vi "nchFFT.vi"(4 "1ch":dbl[](array[numeric]) caption="X1", 5 "频率":dbl) -> (0 "频谱图":dbl[](graph), 2 "幅度值1":dbl)   [LabVIEW 2014]
uses:
  <vilib>/Analysis/2dsp.llb/Real FFT.vi
  <vilib>/Analysis/NI_AALPro.lvlib
panel:
  in  "8ch":dbl[](array[numeric]) caption="X8"
  out "幅度值8":dbl
  out "频谱图 8":dbl[](graph)
  in  "7ch":dbl[](array[numeric]) caption="X7"
  out "幅度值7":dbl
  out "频谱图 7":dbl[](graph)
  in  "6ch":dbl[](array[numeric]) caption="X6"
  out "幅度值6":dbl
  out "频谱图 6":dbl[](graph)
  in  "5ch":dbl[](array[numeric]) caption="X5"
  out "幅度值5":dbl
  out "频谱图 5":dbl[](graph)
  in  "4ch":dbl[](array[numeric]) caption="X4"
  out "幅度值4":dbl
  out "频谱图 4":dbl[](graph)
  in  "3ch":dbl[](array[numeric]) caption="X3"
  out "幅度值3":dbl
  out "频谱图 3":dbl[](graph)
  in  "2ch":dbl[](array[numeric]) caption="X2"
  out "幅度值2":dbl
  out "频谱图 2":dbl[](graph)
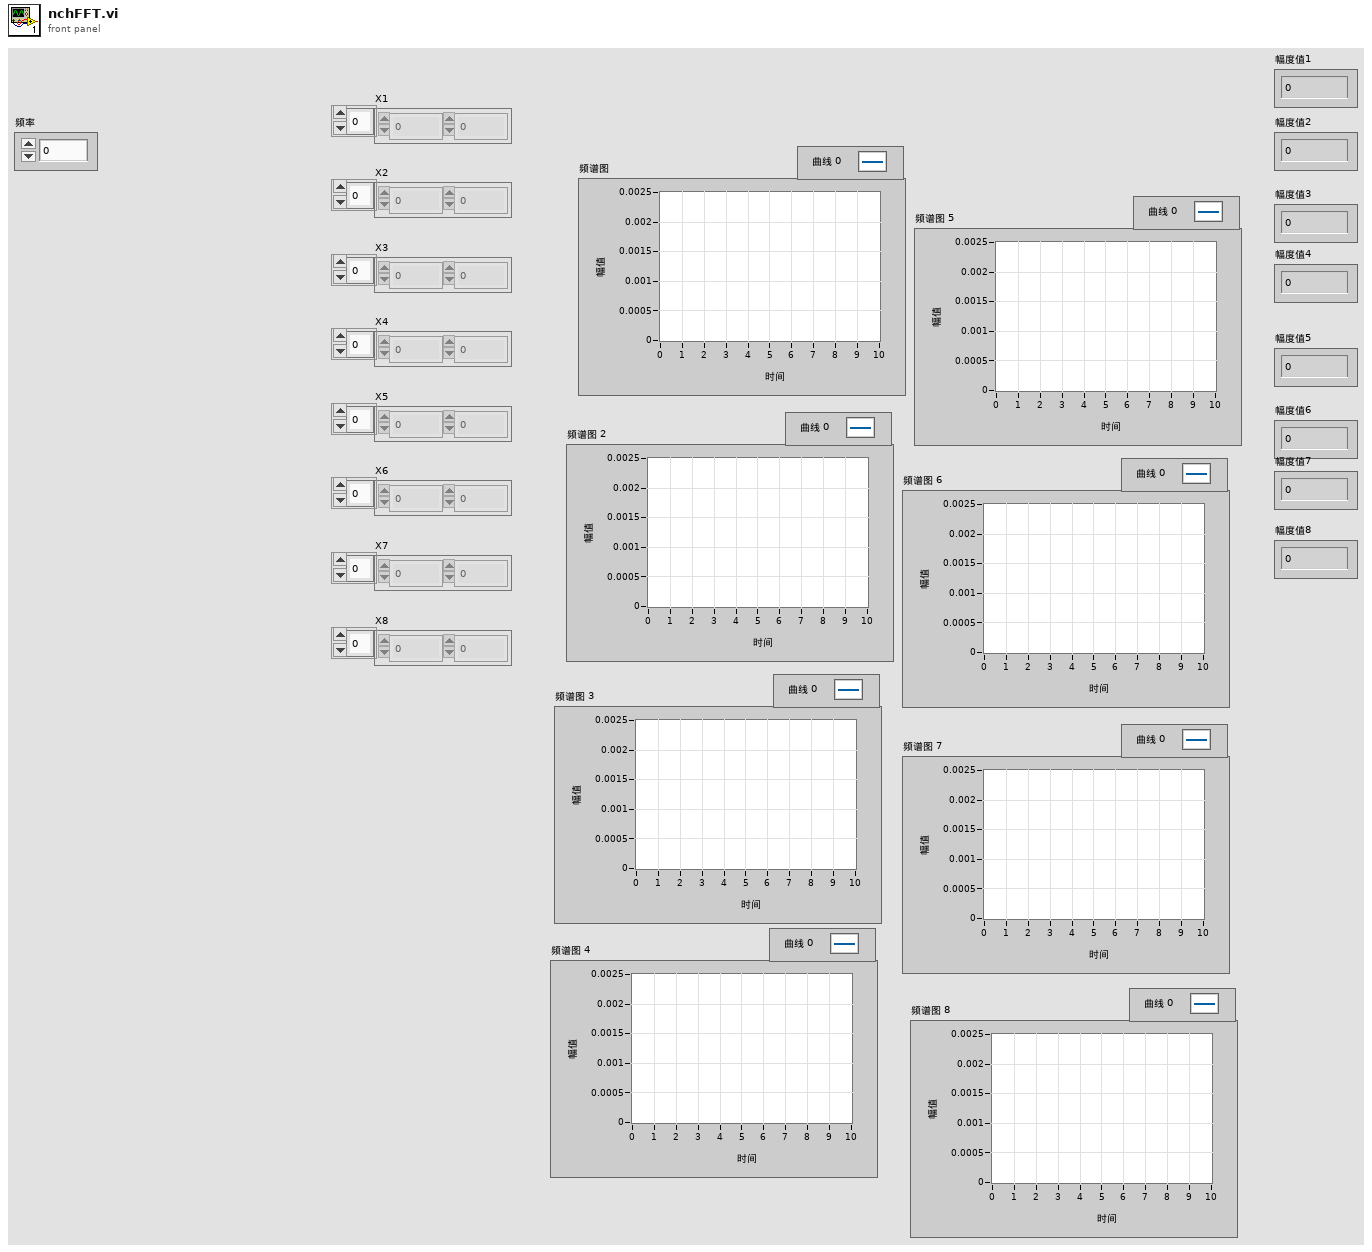
[diagram p1: front panel]
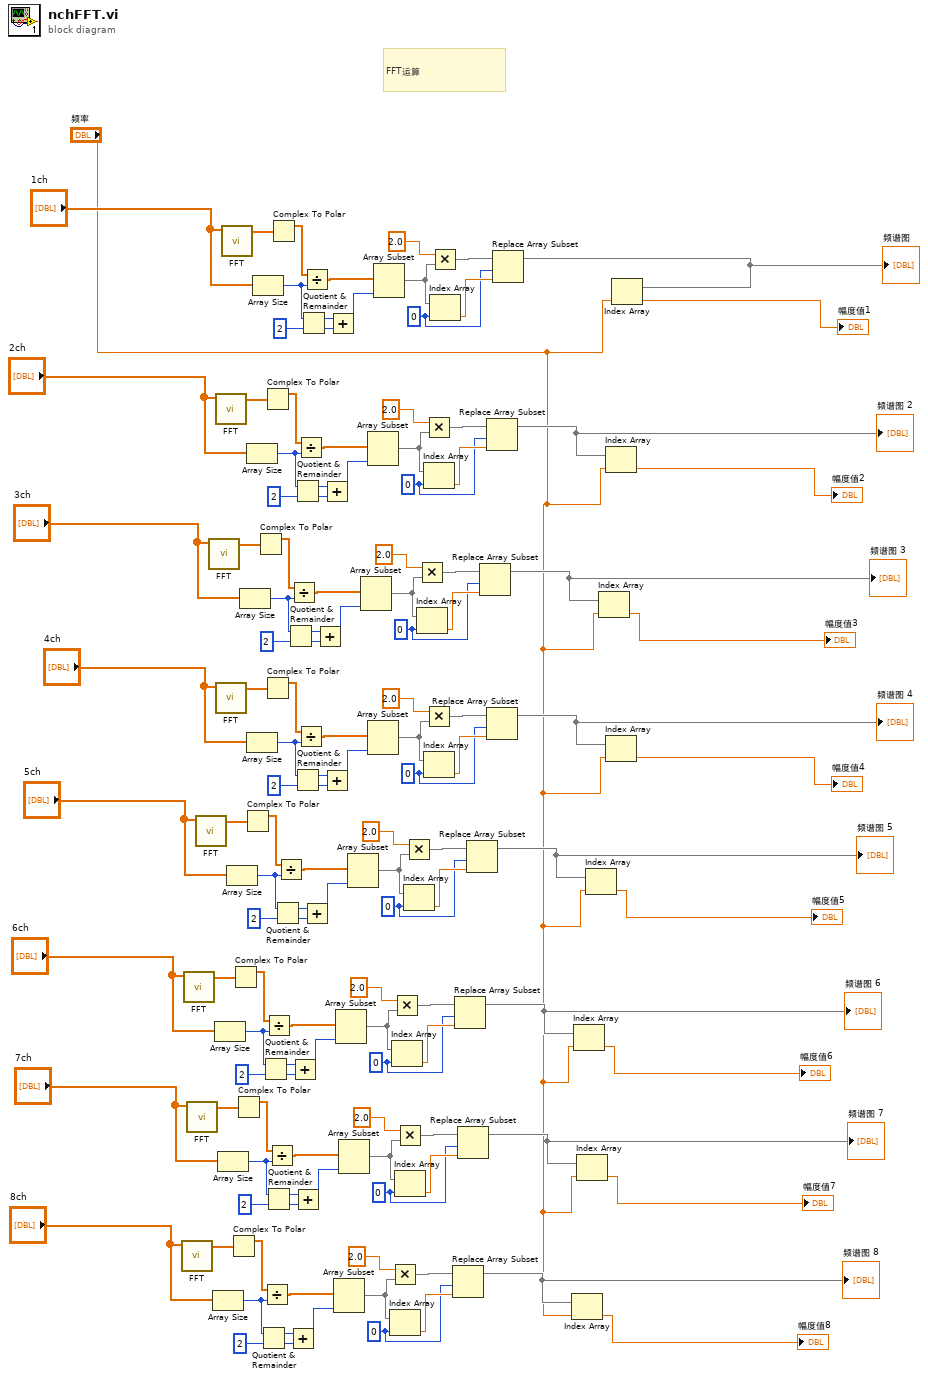
[diagram p0: block diagram]
diagram:
  w8 = 0 ("索引")
  w24 = 0 ("索引")
  w40 = 0 ("索引")
  w56 = 0 ("索引")
  w72 = 0 ("索引")
  w88 = 0 ("索引")
  w104 = 0 ("索引")
  w120 = 0 ("索引")
  # "FFT运算"
  n1 = call-poly <vilib>:"FFT.vi"("X"="8ch") -> ("FFT {X}"=w17:cdb[])  [unwired: 9 in, 1 out]
  n2 = call-poly <vilib>:"FFT.vi"("X"="6ch") -> ("FFT {X}"=w49:cdb[])  [unwired: 9 in, 1 out]
  n3 = call-poly <vilib>:"FFT.vi"("X"="7ch") -> ("FFT {X}"=w33:cdb[])  [unwired: 9 in, 1 out]
  n4 = call-poly <vilib>:"FFT.vi"("X"="5ch") -> ("FFT {X}"=w65:cdb[])  [unwired: 9 in, 1 out]
  n5 = call-poly <vilib>:"FFT.vi"("X"="3ch") -> ("FFT {X}"=w97:cdb[])  [unwired: 9 in, 1 out]
  n6 = Array Size(array="8ch") -> (size(s)=w6:i32)
  n7 = Array Size(array="6ch") -> (size(s)=w38:i32)
  n8 = call-poly <vilib>:"FFT.vi"("X"="2ch") -> ("FFT {X}"=w113:cdb[])  [unwired: 9 in, 1 out]
  n9 = call-poly <vilib>:"FFT.vi"("X"="4ch") -> ("FFT {X}"=w81:cdb[])  [unwired: 9 in, 1 out]
  n10 = Array Size(array="7ch") -> (size(s)=w22:i32)
  n11 = call-poly <vilib>:"FFT.vi"("X"="1ch") -> ("FFT {X}"=w129:cdb[])  [unwired: 9 in, 1 out]
  n12 = Array Size(array="5ch") -> (size(s)=w54:i32)
  n13 = Complex To Polar(r * e^(i*theta)=w17) -> (r=w16:dbl[])  [unwired: 1 out]
  n14 = Complex To Polar(r * e^(i*theta)=w49) -> (r=w48:dbl[])  [unwired: 1 out]
  n15 = Complex To Polar(r * e^(i*theta)=w33) -> (r=w32:dbl[])  [unwired: 1 out]
  n16 = Array Size(array="3ch") -> (size(s)=w86:i32)
  n17 = Complex To Polar(r * e^(i*theta)=w65) -> (r=w64:dbl[])  [unwired: 1 out]
  n18 = Array Size(array="2ch") -> (size(s)=w102:i32)
  n19 = Array Size(array="4ch") -> (size(s)=w70:i32)
  n20 = Array Size(array="1ch") -> (size(s)=w118:i32)
  n21 = Complex To Polar(r * e^(i*theta)=w97) -> (r=w96:dbl[])  [unwired: 1 out]
  n22 = Quotient & Remainder(x=w6, y=2) -> (x-y*floor(x/y)=w14:i32, floor(x/y)=w15:i32)
  n23 = Quotient & Remainder(x=w38, y=2) -> (x-y*floor(x/y)=w46:i32, floor(x/y)=w47:i32)
  n24 = Divide(x=w16, y=w6) -> (x/y=w7:dbl[])
  n25 = Complex To Polar(r * e^(i*theta)=w113) -> (r=w112:dbl[])  [unwired: 1 out]
  n26 = Complex To Polar(r * e^(i*theta)=w81) -> (r=w80:dbl[])  [unwired: 1 out]
  n27 = Divide(x=w48, y=w38) -> (x/y=w39:dbl[])
  n28 = Quotient & Remainder(x=w22, y=2) -> (x-y*floor(x/y)=w30:i32, floor(x/y)=w31:i32)
  n29 = Divide(x=w32, y=w22) -> (x/y=w23:dbl[])
  n30 = Complex To Polar(r * e^(i*theta)=w129) -> (r=w128:dbl[])  [unwired: 1 out]
  n31 = Quotient & Remainder(x=w54, y=2) -> (x-y*floor(x/y)=w62:i32, floor(x/y)=w63:i32)
  n32 = Divide(x=w64, y=w54) -> (x/y=w55:dbl[])
  n33 = Quotient & Remainder(x=w86, y=2) -> (x-y*floor(x/y)=w94:i32, floor(x/y)=w95:i32)
  n34 = Add(x=w14, y=w15) -> (x+y=w13:i32)
  n35 = Divide(x=w96, y=w86) -> (x/y=w87:dbl[])
  n36 = Add(x=w46, y=w47) -> (x+y=w45:i32)
  n37 = Quotient & Remainder(x=w102, y=2) -> (x-y*floor(x/y)=w110:i32, floor(x/y)=w111:i32)
  n38 = Quotient & Remainder(x=w70, y=2) -> (x-y*floor(x/y)=w78:i32, floor(x/y)=w79:i32)
  n39 = Add(x=w30, y=w31) -> (x+y=w29:i32)
  n40 = Divide(x=w112, y=w102) -> (x/y=w103:dbl[])
  n41 = Divide(x=w80, y=w70) -> (x/y=w71:dbl[])
  n42 = Quotient & Remainder(x=w118, y=2) -> (x-y*floor(x/y)=w126:i32, floor(x/y)=w127:i32)
  n43 = Divide(x=w128, y=w118) -> (x/y=w119:dbl[])
  n44 = Add(x=w62, y=w63) -> (x+y=w61:i32)
  n45 = Add(x=w94, y=w95) -> (x+y=w93:i32)
  n46 = Add(x=w110, y=w111) -> (x+y=w109:i32)
  n47 = Add(x=w78, y=w79) -> (x+y=w77:i32)
  n48 = Add(x=w126, y=w127) -> (x+y=w125:i32)
  n49 = Array Subset(array=w7, length=w13) -> (w11:dbl[])  [unwired: 1 in]
  n50 = Array Subset(array=w39, length=w45) -> (w43:dbl[])  [unwired: 1 in]
  n51 = Array Subset(array=w23, length=w29) -> (w27:dbl[])  [unwired: 1 in]
  n52 = Array Subset(array=w55, length=w61) -> (w59:dbl[])  [unwired: 1 in]
  n53 = Array Subset(array=w87, length=w93) -> (w91:dbl[])  [unwired: 1 in]
  n54 = Array Subset(array=w103, length=w109) -> (w107:dbl[])  [unwired: 1 in]
  n55 = Array Subset(array=w71, length=w77) -> (w75:dbl[])  [unwired: 1 in]
  n56 = Array Subset(array=w119, length=w125) -> (w123:dbl[])  [unwired: 1 in]
  n57 = Multiply(x=2.0, y=w11) -> (x*y=w9:dbl[])
  n58 = Index Array(array=w11, index=w8) -> (element=w10:dbl)
  n59 = Multiply(x=2.0, y=w43) -> (x*y=w41:dbl[])
  n60 = Index Array(array=w43, index=w40) -> (element=w42:dbl)
  n61 = Multiply(x=2.0, y=w27) -> (x*y=w25:dbl[])
  n62 = Index Array(array=w27, index=w24) -> (element=w26:dbl)
  n63 = Multiply(x=2.0, y=w59) -> (x*y=w57:dbl[])
  n64 = Index Array(array=w59, index=w56) -> (element=w58:dbl)
  n65 = Multiply(x=2.0, y=w91) -> (x*y=w89:dbl[])
  n66 = Index Array(array=w91, index=w88) -> (element=w90:dbl)
  n67 = Multiply(x=2.0, y=w107) -> (x*y=w105:dbl[])
  n68 = Index Array(array=w107, index=w104) -> (element=w106:dbl)
  n69 = Multiply(x=2.0, y=w75) -> (x*y=w73:dbl[])
  n70 = Index Array(array=w75, index=w72) -> (element=w74:dbl)
  n71 = Multiply(x=2.0, y=w123) -> (x*y=w121:dbl[])
  n72 = Index Array(array=w123, index=w120) -> (element=w122:dbl)
  n73 = Replace Array Subset(array=w9, new element=w10, index=w8) -> (w4:dbl[])
  "频谱图 8" <- w4
  n74 = Replace Array Subset(array=w41, new element=w42, index=w40) -> (w36:dbl[])
  "频谱图 6" <- w36
  n75 = Replace Array Subset(array=w25, new element=w26, index=w24) -> (w20:dbl[])
  "频谱图 7" <- w20
  n76 = Replace Array Subset(array=w57, new element=w58, index=w56) -> (w52:dbl[])
  "频谱图 5" <- w52
  n77 = Replace Array Subset(array=w89, new element=w90, index=w88) -> (w84:dbl[])
  "频谱图 3" <- w84
  n78 = Replace Array Subset(array=w105, new element=w106, index=w104) -> (w100:dbl[])
  "频谱图 2" <- w100
  n79 = Replace Array Subset(array=w73, new element=w74, index=w72) -> (w68:dbl[])
  "频谱图 4" <- w68
  n80 = Replace Array Subset(array=w121, new element=w122, index=w120) -> (w116:dbl[])
  "频谱图" <- w116
  n81 = Index Array(array=w4, index="频率") -> (element=→"幅度值8":dbl)
  n82 = Index Array(array=w36, index="频率") -> (element=→"幅度值6":dbl)
  n83 = Index Array(array=w20, index="频率") -> (element=→"幅度值7":dbl)
  n84 = Index Array(array=w52, index="频率") -> (element=→"幅度值5":dbl)
  n85 = Index Array(array=w84, index="频率") -> (element=→"幅度值3":dbl)
  n86 = Index Array(array=w100, index="频率") -> (element=→"幅度值2":dbl)
  n87 = Index Array(array=w68, index="频率") -> (element=→"幅度值4":dbl)
  n88 = Index Array(array=w116, index="频率") -> (element=→"幅度值1":dbl)
